vi "WILT Add val to Array w Limit.vi"(8 "size limit":i32=26, 9 "Value":dbl, 10 "Array In":dbl[](array[numeric]), 11 "Init?":bool) -> (2 "Array  Out":dbl[](array[numeric]))   [LabVIEW 2016]
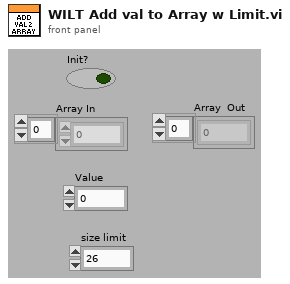
[diagram p1: front panel]
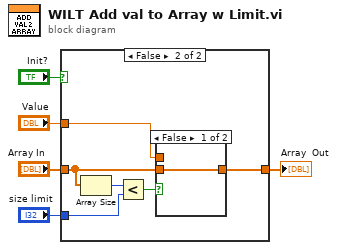
[diagram p0: block diagram]
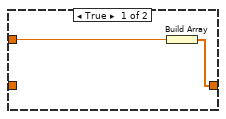
[diagram p2: hidden frame]
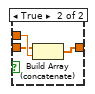
[diagram p3: hidden frame]
diagram:
  n1 = case shown="False" "Init?" {
    tunnel: "Value" -> [w7 w13]
    tunnel: [w6 w12] -> w5
    tunnel: "Array In" -> [_ w11]
    tunnel: "size limit" -> [_ w9]
    frame True {
      n2 = Build Array(w7) -> (w6:dbl[])
    }
    frame False {
      n3 = Array Size(array=w11) -> (size(s)=w10:i32)
      n4 = Less?(x=w10, y=w9) -> (x < y?=w8:bool)
      n5 = case shown="False" w8 {
        tunnel: w13 -> [_ w17]
        tunnel: [w14 w16] -> w12
        tunnel: w11 -> [w14 w15]
        frame False {
        }
        frame True {
          n6 = Build Array (concatenate)(w15, w17) -> (w16:dbl[])
        }
      }
    }
  }
  "Array  Out" <- w5
